vi "Write Flashcards Data.vi"(0 "Write to CSV(T) MDB(F)":bool, 2 "stripped path":path, 12 "Seating Information":T1(array[cluster]), 13 "Color Info":i32[][][](array[numeric])) -> ()   [LabVIEW 2019, in "flashcards.lvlib"]
uses:
  flashcards.lvlib
  Colors.ctl
  <vilib>/Utility/error.llb/DialogType.ctl
panel:
  out "Progress 2":dbl format="%.2f"
  out "Progress":dbl format="%.2f"
  in  "Color":u16(ring)=6 items=["Black", "White", "Orange", "Red", "Blue", "Green", "Disabled"]
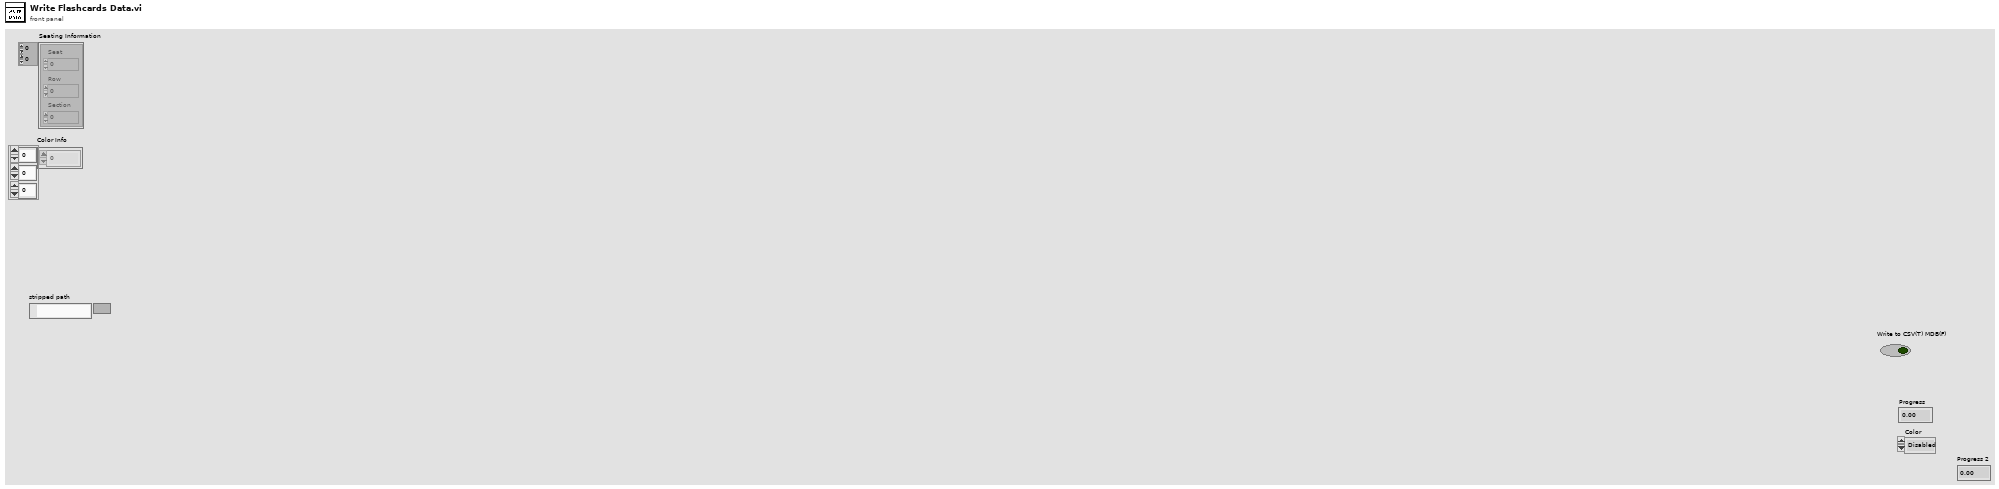
[diagram p1: front panel]
types:
  T1 = cluster{"Seat":i32, "Row":i32, "Section":i32}[][]
  T2 = typedef "flashcards.lvlib/Colors.ctl" = enum16{"Black", "White", "Orange", "Red", "Blue", "Green", "None"}
  T3 = cluster{"[0]":string, "[1]":string, "[2]":string, "[3]":string, "[4]":string, "[5]":string, "[6]":string, "[7]":string, "[8]":string}
  T4 = cluster{string, string, string, "[0]":string, "[1]":string, "[2]":string, "[3]":string, "[4]":string, "[5]":string}
  T5 = typedef "DialogType.ctl" = u16
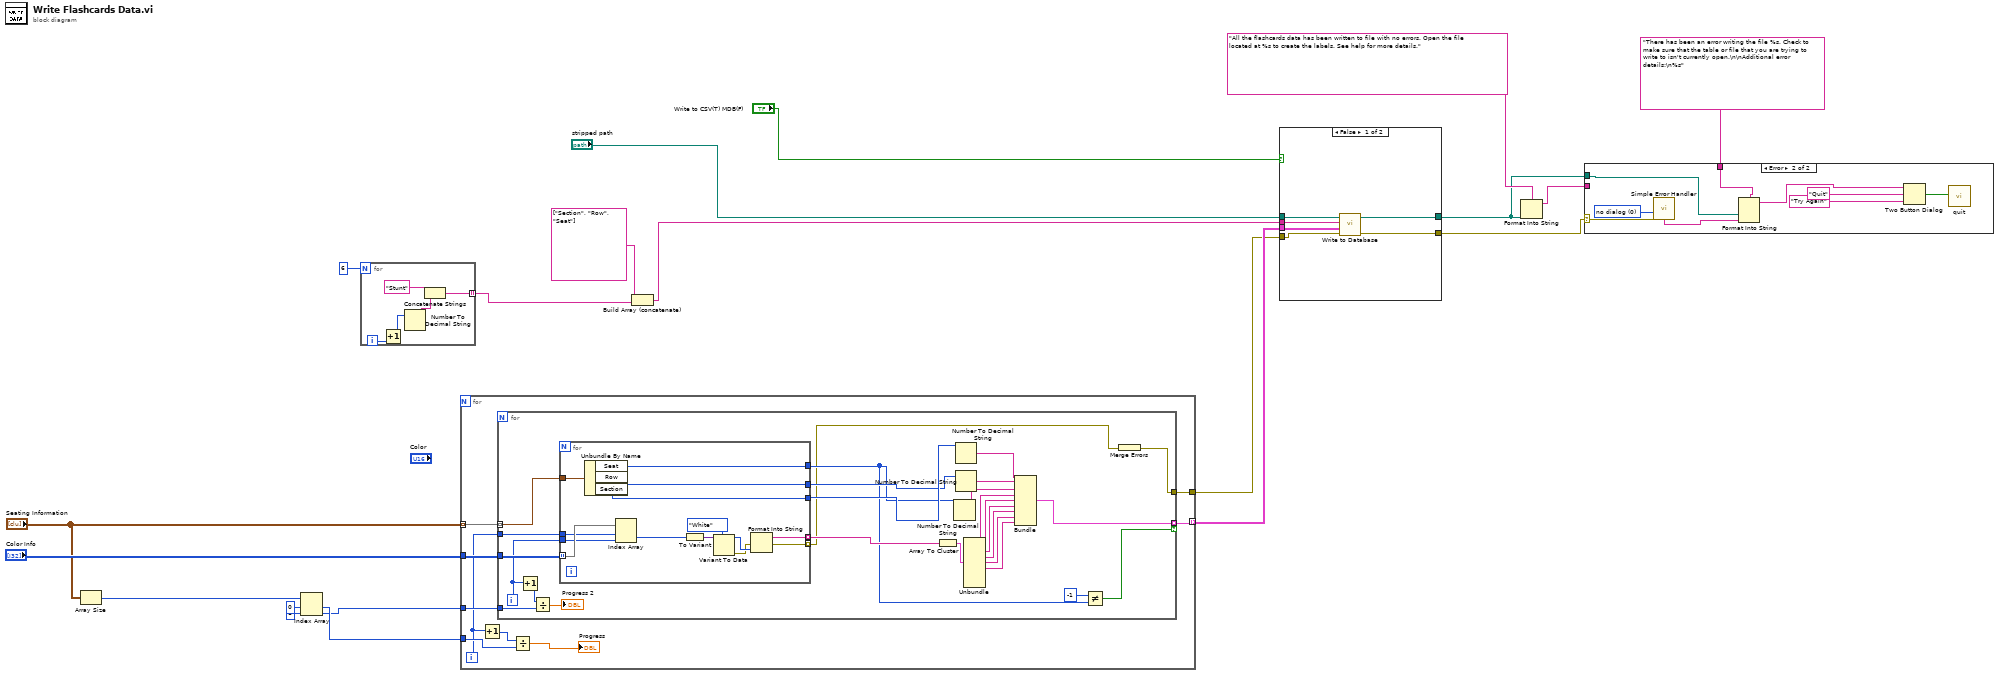
[diagram p0: block diagram]
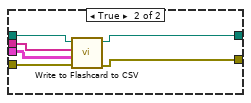
[diagram p2: hidden frame]
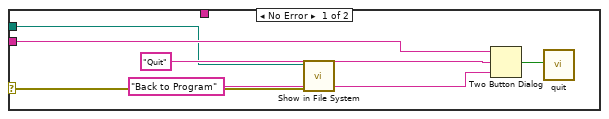
[diagram p3: hidden frame]
diagram:
  n1 = Array Size(array="Seating Information") -> (size(s)=w15:i32[])
  n2 = Index Array(array=w15, index #1=0 ("index"), index #2=1 ("index")) -> (element #1=w13:i32, element #2=w11:i32)
  n3 = for {
    N: 6 -> [_]
    tunnel: [w21] -> w6 mode=indexing
    i -> [w25]
    n4 = Increment(x=w25) -> (x+1=w22:i32)
    n5 = Number To Decimal String(number=w22) -> (decimal integer string=w23:string)  [unwired: 1 in]
    n6 = Concatenate Strings("Stunt", w23) -> (w21:string)
  }
  n7 = for {
    tunnel: [w34] -> w4
    tunnel: "Seating Information" -> [w33] mode=indexing
    tunnel: "Color Info" -> [w32]
    tunnel: w13 -> [w31]
    tunnel: w11 -> [w29]
    tunnel: [w26] -> w9 mode=indexing
    i -> [w28]
    n8 = Increment(x=w28) -> (x+1=w27:i32)
    n9 = for {
      tunnel: [w47] -> w34
      tunnel: w33 -> [w60] mode=indexing
      tunnel: w32 -> [w59]
      tunnel: w28 -> [w58]
      tunnel: w29 -> [w54]
      tunnel: [w46] -> w26 mode=indexing if=w35
      i -> [w52]
      n10 = Increment(x=w52) -> (x+1=w51:i32)
      n11 = Divide(x=w51, y=w54) -> (x/y=→"Progress 2":dbl)
      n12 = for {
        tunnel: w60 -> [w74]
        tunnel: w59 -> [w73] mode=indexing
        tunnel: w58 -> [w72]
        tunnel: w52 -> [w71]
        tunnel: [w70] -> w57
        tunnel: [w69] -> w56
        tunnel: [w68] -> w50
        tunnel: [w63] -> w55 mode=indexing
        tunnel: [w62] -> w48 mode=indexing
        n13 = Unbundle By Name(w74) -> ("Seat"=w68:i32, "Row"=w69:i32, "Section"=w70:i32)
        n14 = Index Array(array=w73, index (row)=w72, index (col)=w71) -> (element=w66:i32)
        n15 = To Variant(anything=w66) -> (Variant=w67:variant)
        n16 = Variant To Data(type=Colors."White" ("Color"), Variant=w67) -> (data=w64:T2, error out=w61:errorcluster)  [unwired: 1 in]
        n17 = Format Into String(error in=w61, w64) -> (resulting string=w63:string, error out=w62:errorcluster)  [unwired: 2 in]
      }
      n18 = Array To Cluster(array=w55) -> (cluster=w42:T3)
      n19 = Number To Decimal String(number=w50) -> (decimal integer string=w43:string)  [unwired: 1 in]
      n20 = Number To Decimal String(number=w57) -> (decimal integer string=w45:string)  [unwired: 1 in]
      n21 = Number To Decimal String(number=w56) -> (decimal integer string=w44:string)  [unwired: 1 in]
      n22 = Unbundle(w42) -> ("[0]"=w41:string, "[1]"=w40:string, "[2]"=w39:string, "[3]"=w38:string, "[4]"=w37:string, "[5]"=w36:string)  [unwired: 3 out]
      n23 = Bundle(w45, w44, w43, "[0]"=w41, "[1]"=w40, "[2]"=w39, "[3]"=w38, "[4]"=w37, "[5]"=w36) -> (w46:T4)  [unwired: 1 in]
      n24 = Not Equal?(x=-1, y=w50) -> (x != y?=w35:bool)
      n25 = Merge Errors(w48) -> (w47:errorcluster)
    }
    n26 = Divide(x=w27, y=w31) -> (x/y=→"Progress":dbl)
  }
  n27 = Build Array (concatenate)(string[] ["Section", "Row", "Seat"], w6) -> (w7:string[])
  n28 = case shown="False" "Write to CSV(T) MDB(F)" {
    tunnel: [w80 w82] -> w18
    tunnel: "stripped path" -> [w79 w85]
    tunnel: w9 -> [w78 w83]
    tunnel: w7 -> [w77 w84]
    tunnel: w4 -> [w76 w86]
    tunnel: [w75 w81] -> w1
    frame False {
      n29 = call "Write to Database.vi"("error in"=w76, "Array 2"=w78, "Array"=w77, "stripped path"=w79) -> ("error out"=w80:errorcluster, "appended path"=w75:path)  [unwired: 5 in, 1 out]
    }
    frame True {
      n30 = call "Write to Flashcard to CSV.vi"("error in"=w86, "DATA"=w83, "Columns"=w84, "stripped path"=w85) -> ("error out"=w82:errorcluster, "actual path"=w81:path)  [unwired: 6 in]
    }
  }
  n31 = Format Into String(format string="All the flashcards data has been written to file with no errors. Open the file located at %s to create the labels. See help for more details." ("message"), w1) -> (resulting string=w2:string)  [unwired: 2 in, 1 out]
  n32 = case shown="Error" w18 {
    selector: w18 -> [w88 w96]
    tunnel: "There has been an error writing the file %s. Check to make sure that the table or file that you are trying to write to isn't currently open.\n\nAdditional error details:\n%s" ("message") -> [_ w98]
    tunnel: w2 -> [w89 _]
    tunnel: w1 -> [w87 w97]
    frame No Error {
      n33 = call <vilib>:"Show in File System.vi"("error in (no error)"=w88, "file or directory path"=w87) -> ()  [unwired: 9 in, 1 out]
      n34 = Two Button Dialog(message=w89, 1:"Back to Program" ("F button name (\"Cancel\")"), 2:"Quit" ("T button name (\"OK\")")) -> (T button?=w90:bool)
      n35 = call "quit.vi"("quit?"=w90) -> ()
    }
    frame Error {
      w95 = T5 0 items=["no dialog", "OK message", "continue or stop message", "OK message + warnings", "continue/stop + warnings"] ("type of dialog (OK msg:1)")
      n36 = call <vilib>:"Simple Error Handler.vi"("type of dialog (OK msg:1)"=w95, "error in (no error)"=w96) -> ("message"=w94:string)  [unwired: 3 in, 4 out]
      n37 = Format Into String(format string=w98, w97, w94) -> (resulting string=w93:string)  [unwired: 2 in, 1 out]
      n38 = Two Button Dialog(message=w93, 1:"Try Again" ("F button name (\"Cancel\")"), 2:"Quit" ("T button name (\"OK\")")) -> (T button?=w99:bool)
      n39 = call "quit.vi"("quit?"=w99) -> ()
    }
  }
